vi "FormCalibra.vi"() -> ()   [LabVIEW 2014]
panel:
  out "Temperature 2 (degC)":dbl
  out "Temperature 1 (degC)":dbl
  out "Emf (Thermo 2 - mV)":dbl
  out "Emf (Thermo 1 - mV)":dbl
  out "Emf (Hot Temp 2 - mV)":dbl
  out "Input Voltage Thermo 2 (V)":dbl
  out "Input Voltage Thermo 1 (V)":dbl
  out "Emf (Hot Temp 1 - mV)":dbl
  out "Emf (Cold - mV)":dbl
  out "Temperature Ref (degC)":dbl
  # "Temperatura da junta fria"
  # "Temperatura termopares"
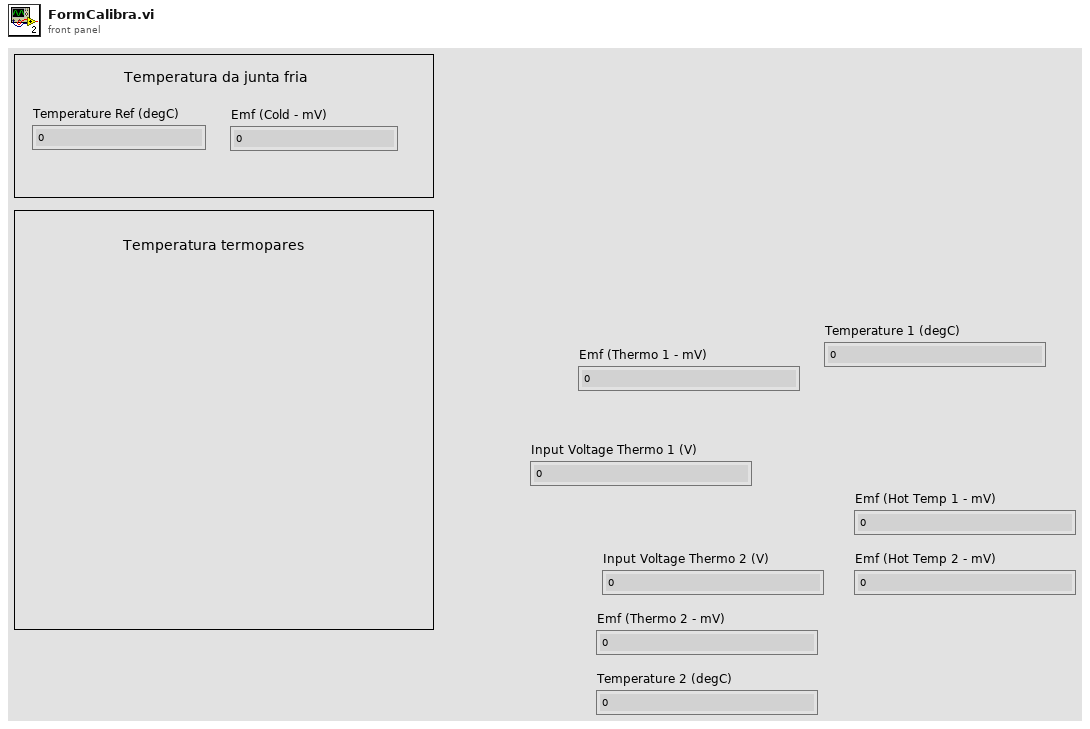
[diagram p1: front panel]
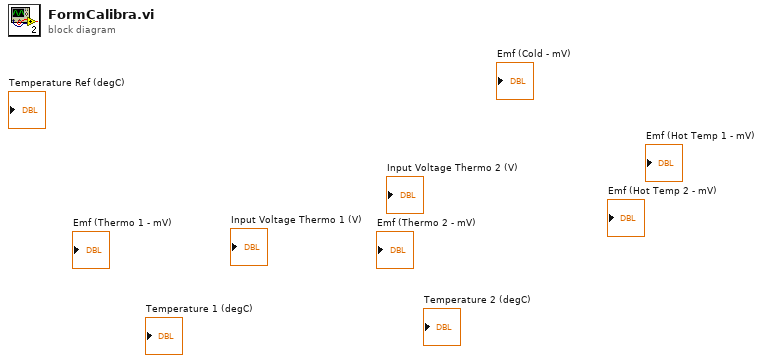
[diagram p0: block diagram]
diagram:
